vi "Get Strain.vi"(6 "Channel":i32=1 min=1 max=2, 8 "error in (no error)":errorcluster, 11 "Inst.RP100 in":refnum<class "Inst.RP100.lvclass">) -> (0 "error out":errorcluster, 2 "Strain (Ch1) (V)":dbl, 3 "Inst.RP100 out":refnum<class "Inst.RP100.lvclass">)   [LabVIEW 2019, in "Inst.RP100.lvclass"]
uses:
  Inst.RP100.lvclass
  C:/Program Files (x86)/National Instruments/LabVIEW 2019/user.lib/LevyLab/Instrument Framework/SMOs/Instrument/Instrument.lvclass
  Typedefs/Commands--Enum.ctl
  <userlib>/LevyLab/Instrument Framework/SMOs/Instrument/Instrument.lvclass/Instrument.ctl
  6b62cf6d-5fa0-488a-a9a9-66311bb438ee.vi
  6b62cf6d-5fa0-488a-a9a9-66311bb438ee.vi/df89f6ce-8bff-4edb-b5cf-9975733845e1.vi
  6b62cf6d-5fa0-488a-a9a9-66311bb438ee.vi/df89f6ce-8bff-4edb-b5cf-9975733845e1.vi/c61f8c22-9c30-4ac6-8982-aa6faf893cbc.vi
  <userlib>/LevyLab/Instrument Framework/SMOs/Instrument/API/Send and Receive.vi
  6b62cf6d-5fa0-488a-a9a9-66311bb438ee.vi/df89f6ce-8bff-4edb-b5cf-9975733845e1.vi/c446c6ae-ecac-44db-b096-4502618def96.vi
  <userlib>/LevyLab/Instrument Framework/SMOs/Instrument/Private/Get Client Type.vi
  6b62cf6d-5fa0-488a-a9a9-66311bb438ee.vi/df89f6ce-8bff-4edb-b5cf-9975733845e1.vi/c61f8c22-9c30-4ac6-8982-aa6faf893cbc.vi/4721c5ba-6569-4546-b473-6a63f9449ec2.vi
  6b62cf6d-5fa0-488a-a9a9-66311bb438ee.vi/df89f6ce-8bff-4edb-b5cf-9975733845e1.vi/c61f8c22-9c30-4ac6-8982-aa6faf893cbc.vi/b8196f59-e969-4192-9407-4925a2a5df81.vi
  6b62cf6d-5fa0-488a-a9a9-66311bb438ee.vi/df89f6ce-8bff-4edb-b5cf-9975733845e1.vi/c446c6ae-ecac-44db-b096-4502618def96.vi/5ddbb950-9b3e-4c4a-b4d6-13e8dcdc069a.vi
  6b62cf6d-5fa0-488a-a9a9-66311bb438ee.vi/df89f6ce-8bff-4edb-b5cf-9975733845e1.vi/c446c6ae-ecac-44db-b096-4502618def96.vi/ad8a504a-0b8e-4963-8985-595f5a37ec15.vi
  6b62cf6d-5fa0-488a-a9a9-66311bb438ee.vi/df89f6ce-8bff-4edb-b5cf-9975733845e1.vi/c446c6ae-ecac-44db-b096-4502618def96.vi/5ddbb950-9b3e-4c4a-b4d6-13e8dcdc069a.vi/b5a271cb-3351-4b76-8487-49a9e74b9c6e.vi
  6b62cf6d-5fa0-488a-a9a9-66311bb438ee.vi/df89f6ce-8bff-4edb-b5cf-9975733845e1.vi/c446c6ae-ecac-44db-b096-4502618def96.vi/5ddbb950-9b3e-4c4a-b4d6-13e8dcdc069a.vi/e73d5417-dba7-48e7-8ef9-67f052a4d404.vi
  <userlib>/LevyLab/Instrument Framework/SMOs/Instrument/Private/Get RC Connection Status.vi
  <userlib>/LevyLab/Instrument Framework/SMOs/Instrument/API/Enum to String.vi
  <userlib>/LevyLab/Instrument Framework/SMOs/RemoteControl/API/Send and Receive.vi
  <vilib>/Utility/Data Type/Get Type Information.vi
  <vilib>/JDP Science/JSONtext/JSON text to Variant.vi
  <userlib>/LevyLab/Instrument Framework/SMOs/Instrument/API/Instrument.GetPublicEvents.vi
  <vilib>/JDP Science/JSONtext/Variant to JSON Text.vi
  <vilib>/National Instruments/GUID Generator/Guid Generator.vi
  <userlib>/LevyLab/Instrument Framework/SMOs/Instrument/API/Instrument.MessageToProcess.vi
  <userlib>/LevyLab/Instrument Framework/SMOs/Instrument/Private/Instrument.MessageFromProcess.EventStructure.vi
  <vilib>/JDP Science/JSONtext/LVClass Serializer/JSONtext LVClass Serializer.lvclass
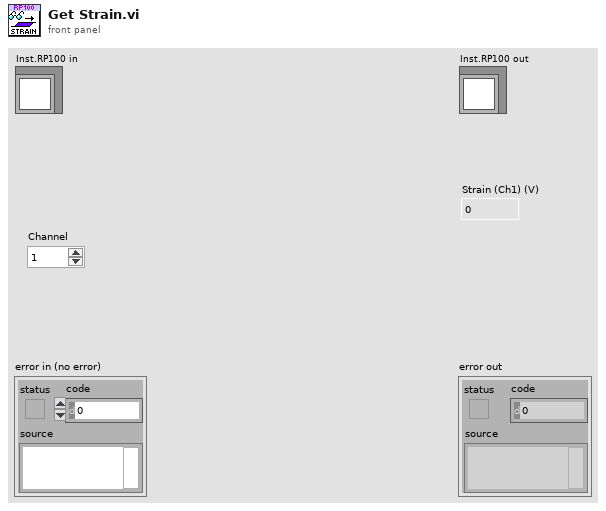
[diagram p1: front panel]
types:
  T1 = typedef "Inst.RP100.lvclass/Commands--Enum.ctl" = enum16{"setState", "setStrain", "getStrain", "setLevel", "getLevel"}
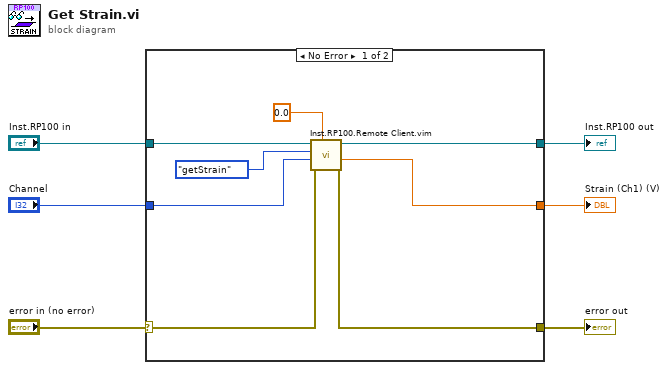
[diagram p0: block diagram]
diagram:
  n1 = case shown="No Error" "error in (no error)" {
    selector: "error in (no error)" -> [w10 w16]
    tunnel: [w9 w16] -> w5
    tunnel: "Inst.RP100 in" -> [w14 w15]
    tunnel: [w13 w15] -> w3
    tunnel: [w7 _] -> w2
    tunnel: "Channel" -> [w11 _]
    frame No Error {
      n2 = call "Inst.RP100.Remote Client.vim"("Data Out type"=0.0 ("Data out"), "error in (no error)"=w10, "params"=w11, "Commands"=Commands--Enum."getStrain", "Inst.RP100 in"=w14) -> ("error out"=w9:errorcluster, "Data out"=w7:dbl, "Inst.RP100 out"=w13:refnum<class "Inst.RP100.lvclass">)  [unwired: 4 in]
    }
    frame Error {
    }
  }
  "error out" <- w5
  "Inst.RP100 out" <- w3
  "Strain (Ch1) (V)" <- w2
